vi "Close View.vi"(8 "error in (no error)":errorcluster, 10 "Hide? (F)":bool, 11 "IViewable in":refnum<class "IViewable.lvclass">) -> (0 "error out":errorcluster, 3 "IViewable out":refnum<class "IViewable.lvclass">)   [LabVIEW 2015, in "IViewable.lvlib" / "IViewable.lvclass"]
doc: "<License>\nCopyright © 2017 Composed Systems, LLC | All rights reserved\nwww.composed.io\n\nAuthor: Ethan Stern <ethan.stern@composed.io>\n\nThis software is provided \"AS IS\" WITHOUT WARRANTIES, either express or implied, AND IS FOR EDUCATIONAL PURPOSES ONLY.\n</License>"
uses:
  IViewable.lvclass
  IViewable.lvclass/IViewable.ctl
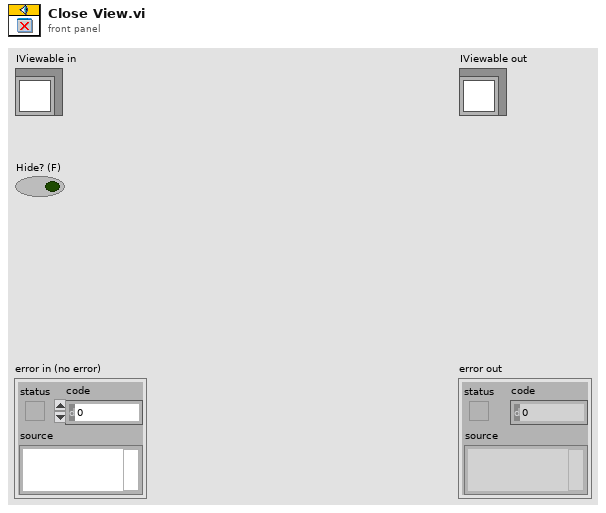
[diagram p1: front panel]
types:
  T1 = enum32{"Invalid", "Standard", "Closed", "Hidden", "Minimized", "Maximized"}
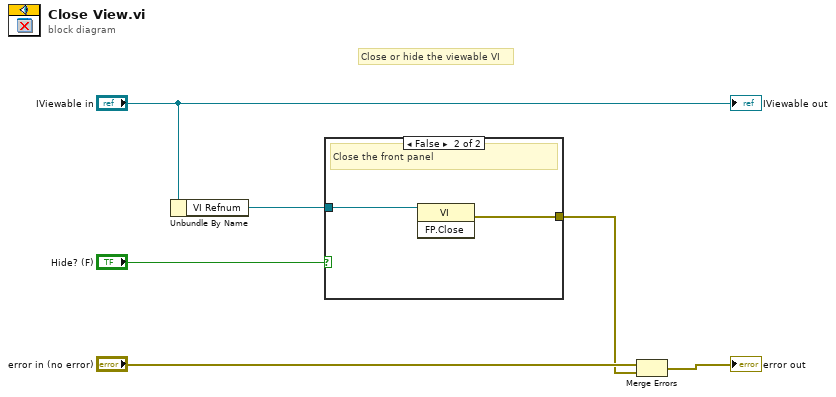
[diagram p0: block diagram]
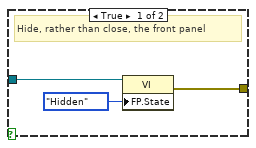
[diagram p2: hidden frame]
diagram:
  # "Close or hide the viewable VI"
  n1 = Unbundle By Name("IViewable in") -> ("VI Refnum"=w2:refnum<vi>)
  n2 = case shown="False" "Hide? (F)" {
    tunnel: [w9 w11] -> w3
    tunnel: w2 -> [w8 w10]
    frame True {
      # "Hide, rather than close, the front panel"
      n3 = property class="VI"(reference=w8, "FP.State"=T1."Hidden" ("Front Panel Window:State")) -> (error out=w9:errorcluster)  [unwired: 1 in, 1 out]
    }
    frame False {
      # "Close the front panel"
      n4 = invoke class="VI" method="FP.Close"(reference=w10) -> (error out=w11:errorcluster)  [unwired: 2 in, 2 out]
    }
  }
  n5 = Merge Errors("error in (no error)", w3) -> (→"error out":errorcluster)
  "IViewable out" <- "IViewable in"
